vi "ExternalInModeList.vi"(10 "List":u32) -> (2 "GetLUTModeList":cluster{string, i32})   [LabVIEW 2015]
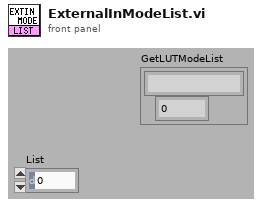
[diagram p1: front panel]
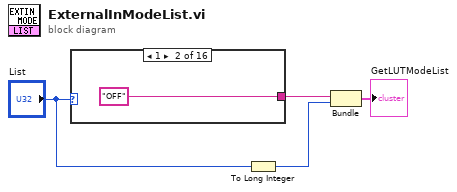
[diagram p0: block diagram]
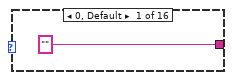
[diagram p2: hidden frame]
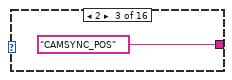
[diagram p3: hidden frame]
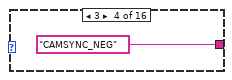
[diagram p4: hidden frame]
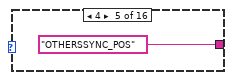
[diagram p5: hidden frame]
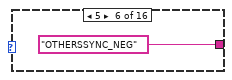
[diagram p6: hidden frame]
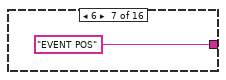
[diagram p7: hidden frame]
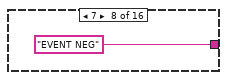
[diagram p8: hidden frame]
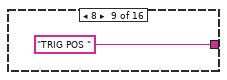
[diagram p9: hidden frame]
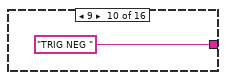
[diagram p10: hidden frame]
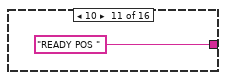
[diagram p11: hidden frame]
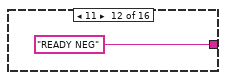
[diagram p12: hidden frame]
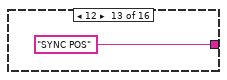
[diagram p13: hidden frame]
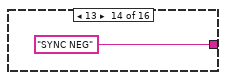
[diagram p14: hidden frame]
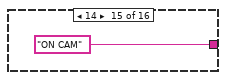
[diagram p15: hidden frame]
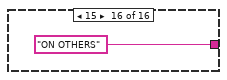
[diagram p16: hidden frame]
diagram:
  n1 = case shown="1" "List" {
    tunnel: ["" "OFF" "CAMSYNC_POS" "CAMSYNC_NEG" "OTHERSSYNC_POS" "OTHERSSYNC_NEG" "EVENT POS" "EVENT NEG" "TRIG POS " "TRIG NEG " "READY POS " "READY NEG" "SYNC POS" "SYNC NEG" "ON CAM" "ON OTHERS"] -> w3
    frame 0, Default {
    }
    frame 1 {
    }
    frame 2 {
    }
    frame 3 {
    }
    frame 4 {
    }
    frame 5 {
    }
    frame 6 {
    }
    frame 7 {
    }
    frame 8 {
    }
    frame 9 {
    }
    frame 10 {
    }
    frame 11 {
    }
    frame 12 {
    }
    frame 13 {
    }
    frame 14 {
    }
    frame 15 {
    }
  }
  n2 = To Long Integer(number="List") -> (32bit integer=w2:i32)
  n3 = Bundle(w3, w2) -> (→"GetLUTModeList":cluster{string, i32})  [unwired: 1 out]
